vi "testErrorMessage.vi"() -> ()   [LabVIEW 2019, in "AssertionTest.lvlib" / "AssertStringContainsString.lvlib"]
uses:
  AssertStringContainsString.lvlib
  Assertion/Assertion.lvlib
panel:
  out "error out":errorcluster
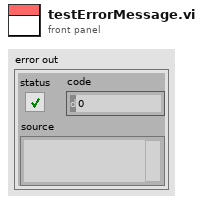
[diagram p1: front panel]
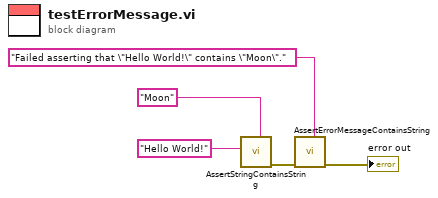
[diagram p0: block diagram]
diagram:
  n1 = call "AssertStringContainsString.vi"("Needle"="Moon", "Haystack"="Hello World!") -> ("error out"=w1:errorcluster)  [unwired: 9 in]
  n2 = call "AssertErrorMessageContainsString.vi"("Expected"="Failed asserting that \"Hello World!\" contains \"Moon\".", "error in (no error)"=w1) -> ("error out"=→"error out":errorcluster)  [unwired: 9 in]
